vi "Calculate INL.vi"(0 "Actual X":dbl[](array[numeric]), 1 "Best Fit?":bool, 5 "Actual Y":dbl[](array[numeric]), 7 "Ideal X":dbl[](array[numeric]), 9 "Ideal Y":dbl[](array[numeric]), 11 "Error in":errorcluster, 12 "ADC?":bool) -> (4 "INL X Plot values":dbl[](array[numeric]), 6 "INL Y Plot Values":dbl[](array[numeric]), 8 "INL Result values":dbl[](array[numeric]), 15 "Error out":errorcluster)   [LabVIEW 2020, in "INL DNL Test.lvclass"]
doc: "Calculates INL result based on bestfit/endpoint method"
uses:
  INL DNL Test.lvclass
  <vilib>/Analysis/6fits.llb/Curve Fitting Criteria.ctl
  <vilib>/Analysis/NI_AALPro.lvlib
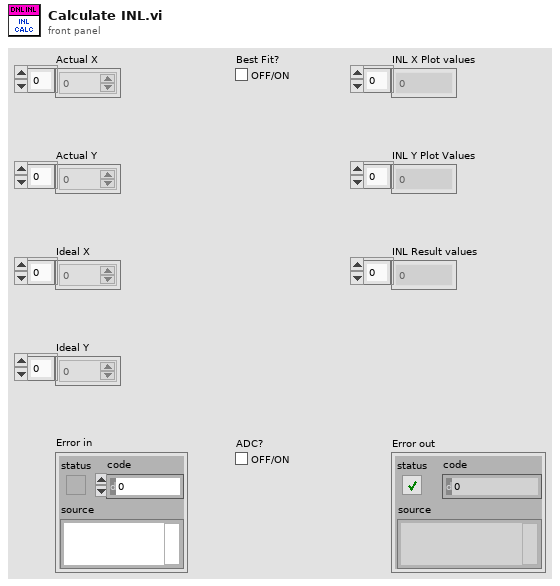
[diagram p1: front panel]
types:
  T1 = typedef "NI_AALPro.lvlib/Curve Fitting Criteria.ctl" = u16
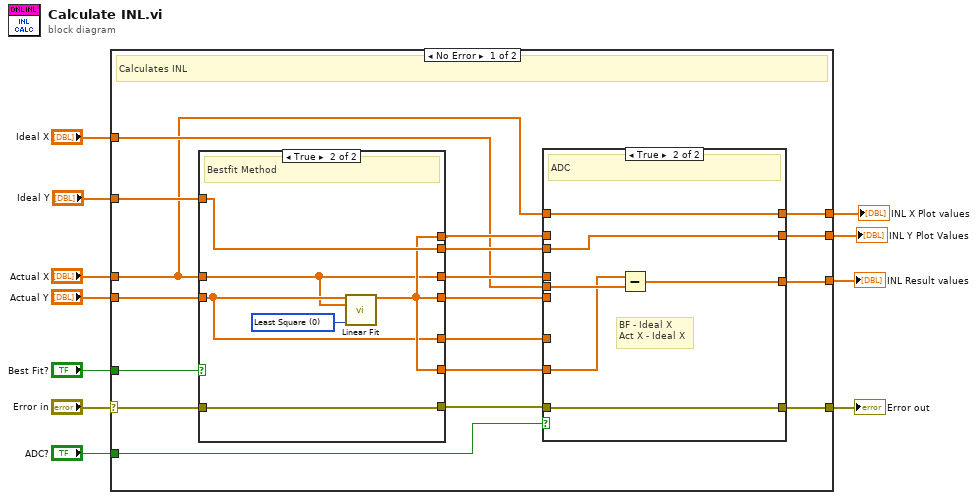
[diagram p0: block diagram]
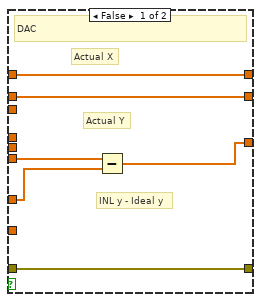
[diagram p3: hidden frame]
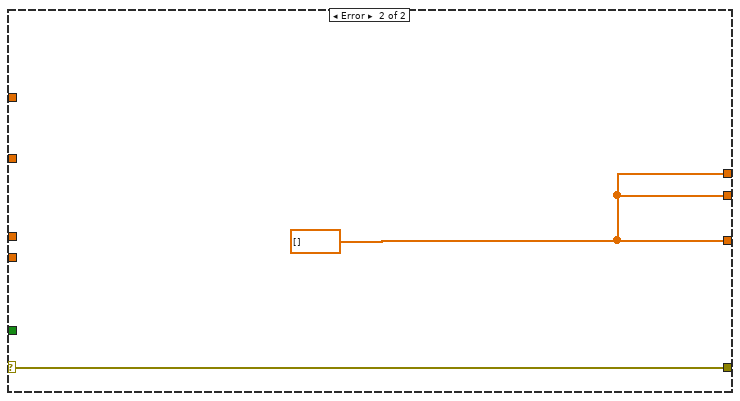
[diagram p4: hidden frame]
diagram:
  n1 = case shown="No Error" "Error in" {
    selector: "Error in" -> [w27 w53]
    tunnel: "Best Fit?" -> [w29 _]
    tunnel: "Actual X" -> [w12 _]
    tunnel: "Actual Y" -> [w28 _]
    tunnel: "Ideal X" -> [w14 _]
    tunnel: "Ideal Y" -> [w16 _]
    tunnel: "ADC?" -> [w26 _]
    tunnel: [w23 w53] -> w3
    tunnel: [w22 w52] -> w4
    tunnel: [w19 w52] -> w2
    tunnel: [w17 w52] -> w1
    frame No Error {
      # "Calculates INL"
      n2 = case shown="True" w29 {
        tunnel: w12 -> [w30 w34]
        tunnel: w28 -> [w31 w35]
        tunnel: [w31 w36] -> w20
        tunnel: [w30 w34] -> w25
        tunnel: w27 -> [w33 w38]
        tunnel: [w33 w38] -> w24
        tunnel: [w32 w35] -> w21
        tunnel: w16 -> [w32 w37]
        tunnel: [w31 w36] -> w18
        tunnel: [w31 w37] -> w15
        tunnel: [w30 w36] -> w13
        frame False {
          # "Endpoint Method"
        }
        frame True {
          w39 = T1 0 items=["Least Square", "Least Absolute Residual", "Bisquare"] ("method")
          # "Bestfit Method"
          n3 = call <vilib>:"Linear Fit.vi"("Y"=w35, "X"=w34, "method"=w39) -> ("Best Linear Fit"=w36:dbl[])  [unwired: 8 in, 4 out]
        }
      }
      n4 = case shown="True" w26 {
        tunnel: w14 -> [_ w50]
        tunnel: w25 -> [_ _]
        tunnel: [w44 w51] -> w22
        tunnel: w20 -> [w45 _]
        tunnel: w24 -> [w43 w49]
        tunnel: [w43 w49] -> w23
        tunnel: w21 -> [w42 _]
        tunnel: w18 -> [w41 _]
        tunnel: [w41 w46] -> w19
        tunnel: w12 -> [w40 w47]
        tunnel: [w40 w47] -> w17
        tunnel: w15 -> [_ w46]
        tunnel: w13 -> [_ w48]
        frame False {
          # "Actual Y"
          # "Actual X"
          # "INL y - Ideal y"
          # "DAC"
          n5 = Subtract(x=w45, y=w42) -> (x-y=w44:dbl[])
        }
        frame True {
          # "BF - Ideal X\nAct X - Ideal X"
          # "ADC"
          n6 = Subtract(x=w48, y=w50) -> (x-y=w51:dbl[])
        }
      }
    }
    frame Error {
      w52 = dbl[] []
    }
  }
  "INL Result values" <- w4
  "Error out" <- w3
  "INL Y Plot Values" <- w2
  "INL X Plot values" <- w1
